vi "Plotting List Box Names.vi"(8 "Error In":errorcluster, 10 "Item Names":string[](array[string]), 11 "Station 1":dbl[][](array[numeric])) -> (0 "Error Out":errorcluster, 2 "time stamp":timestamp, 3 "Listbox names":string[][](array[string]))   [LabVIEW 2016]
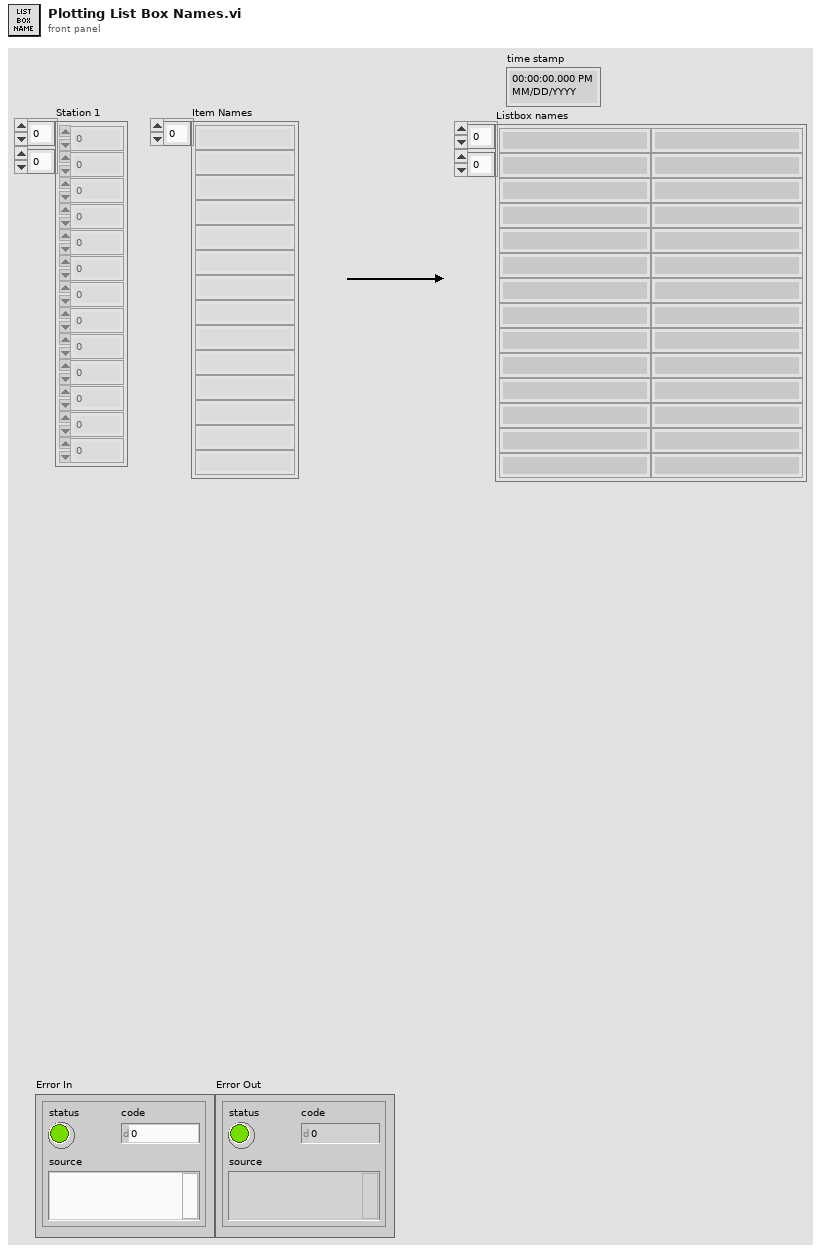
[diagram p1: front panel]
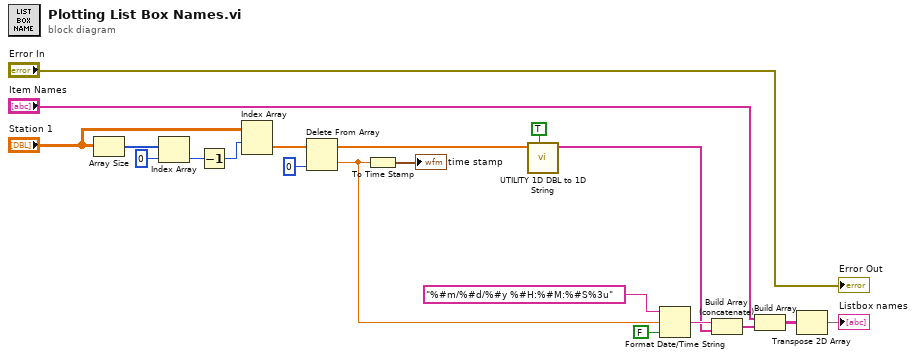
[diagram p0: block diagram]
diagram:
  n1 = Array Size(array="Station 1") -> (size(s)=w2:i32[])
  n2 = Index Array(array=w2, index=0) -> (element=w8:i32)
  n3 = Decrement(x=w8) -> (x-1=w9:i32)
  n4 = Index Array(array="Station 1", index (row)=w9) -> (element=w10:dbl[])  [unwired: 1 in]
  n5 = Delete From Array(array=w10, index=0) -> (deleted portion=w19:dbl, array with subset deleted=w12:dbl[])  [unwired: 1 in]
  n6 = To Time Stamp(1:w19) -> (0:→"time stamp":timestamp)
  n7 = call "UTILITY 1D DBL to 1D String.vi"("DBL?"=TRUE, "1D DBL"=w12) -> ("1D String"=w15:string[])  [unwired: 9 in]
  n8 = Format Date/Time String(time format string (%c)="%#m/%#d/%#y %#H:%#M:%#S%3u", seconds (now)=w19, UTC format=FALSE) -> (date/time string=w16:string)
  n9 = Build Array (concatenate)(w16, w15) -> (w17:string[])
  n10 = Build Array("Item Names", w17) -> (w6:string[][])
  n11 = Transpose 2D Array(2D array=w6) -> (transposed array=→"Listbox names":string[][])
  "Error Out" <- "Error In"
